vi "StaticStrings2_171213.vi"() -> (2 "Port Selection":string, 3 "Display":string, 4 "2":string, 6 "6":string, 8 "Midfield":string, 10 "7":string, 12 "Notifications":string, 13 "1":string, 14 "9":string)   [LabVIEW 2016]
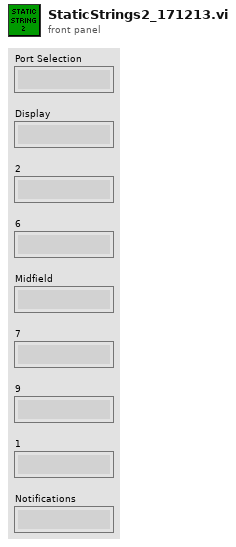
[diagram p1: front panel]
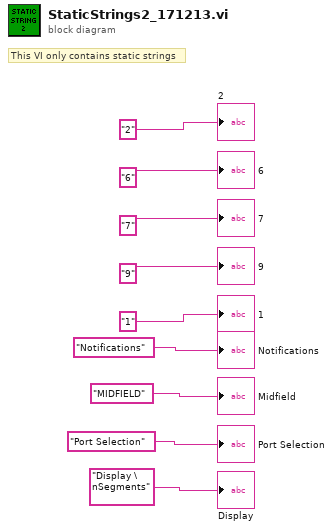
[diagram p0: block diagram]
diagram:
  # "This VI only contains static strings"
  "Notifications" <- "Notifications" ("String 31")
  "Midfield" <- "MIDFIELD" ("String 37")
  "Display" <- "Display \nSegments" ("String 6")
  "1" <- "1" ("String 16")
  "2" <- "2" ("String 15")
  "6" <- "6" ("String 22")
  "7" <- "7" ("String 24")
  "9" <- "9" ("String 25")
  "Port Selection" <- "Port Selection" ("String 33")
